vi "GetIndexArrayReference.vi"(8 "error in":errorcluster, 11 "Index Array in":refnum<class "IndexArray.lvclass">) -> (0 "error out":errorcluster, 1 "reference out":refnum<vi>, 3 "Index Array out":refnum<class "IndexArray.lvclass">)   [LabVIEW 2014, in "IndexArray.lvclass"]
uses:
  IndexArray.lvclass
  Generic/Generic.lvclass
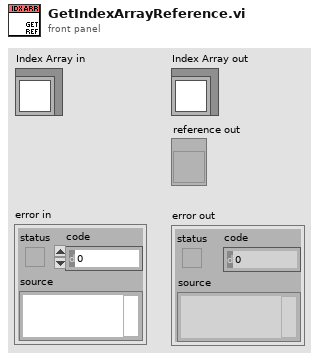
[diagram p1: front panel]
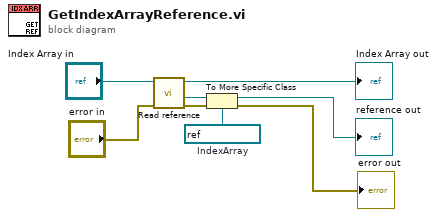
[diagram p0: block diagram]
diagram:
  w8 = refnum<vi> refnum  # IndexArray
  n1 = call "Read reference.vi"("error in"="error in", "GObject in"="Index Array in") -> ("error out"=w7:errorcluster, "reference"=w6:refnum<vi>, "GObject out"=→"Index Array out":refnum<class "IndexArray.lvclass">)  [unwired: 5 in]
  n2 = To More Specific Class(target class=w8, reference=w6, error in=w7) -> (specific class reference=→"reference out":refnum<vi>, error out=→"error out":errorcluster)
